vi "PH_Switch.panel.vi"(0 "object ref":refnum<vi>, 5 "error in (no error)":errorcluster) -> (19 "error out":errorcluster)   [LabVIEW 2014, in "PH_Switch.lvlib"]
doc: "By this VI a hardware switch can be monitored and switched. \n\nThe indicators \"FALSE\", \"TRUE\" and \"SWITCH STATE\" show the value of the Beckhoff-Tag: blue indicates bad tag status reference problems, darkgreen false and lightgreen true. If everything is working fine, \"FALSE\" and \"SWITCH STATE\" should show the same value, while \"TRUE\" has the opposite value. The caption of the sensors for \"FALSE\" and \"TRUE\" are taken out of the database. In case of only one or no sensor these GUI elements are not shown at all.\n\nThe oval button switches. It should be in the same state as the \"SWITCH STATE\" indicator. \n\n\"Delete Instance\" disconnects and removes the instance from the PCS.\n\n\nLicense Agreement for this software:\n\nCopyright (C)\nGesellschaft für Schwerionenforschung, GSI\nPlanckstr. 1\n64291 Darmstadt\nGermany\n\nContact: D.Beck@gsi.de \n\nThis program is free software; you can redistribute it and/or modify it under the terms of the GNU General Public License as published by the Free Software Foundation; either version 2 of the license, or (at your option) any later version.\n\nThis program is distributed in the hope that it will be useful, but WITHOUT ANYW ARRANTY; without even the implied warranty of MERCHANTABILITY or FITNESS FOR A PARTICULAR PURPOSE. See the GNU General License for more details (http://www.gnu.org).\n\nGesellschaft für Schwerionenforschung, GSI\nPlanckstr. 1, 64291 Darmstadt, Germany\nFor all questions and ideas contact: M.Richter@gsi.de, H.Brand@gsi.de or D.Beck@gsi.de.\nLast update: 18-DEC-2002"
uses:
  PH_Switch.lvlib
  PH_StatusHandler/PH_StatusHandler.GUI element.ctl
  PH_Switch.GUI Refs.ctl
  CSCore/CSObj/CSObj.lvlib
  CSCore/CSSystem/CSSystemLib/CSSystemLib.lvlib
  PH_Common/PH_Common.lvlib
  PH_PSDBWriter/PH_PSDBWriter.lvlib
  PH_Class/PH_Class.lvlib
  PH_StatusHandler/PH_StatusHandler.lvlib
panel:
  out "Textfield":string="Testtext"
  out "PSDB Status":u32(colorbox)=6618880 caption="PSDB"
  out "Status":T1 caption="Enabling State"
  in  "Exit":bool
  in  "Delete":bool
  in  "Knob":bool
  out "SW STATE":u32(colorbox)
  out "FALSE":u32(colorbox)
  out "TRUE":u32(colorbox)
  # "PCS"
  # "3.40"
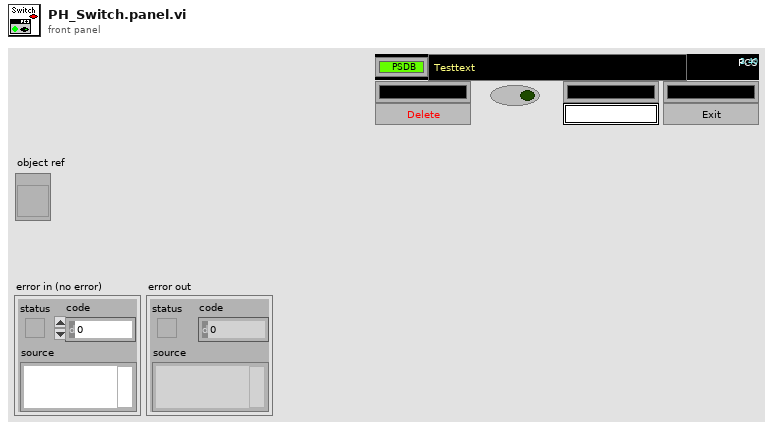
[diagram p1: front panel]
types:
  T1 = typedef "PH_StatusHandler.lvlib/PH_StatusHandler.GUI element.ctl" = u16
  T2 = typedef "PH_Switch.lvlib/PH_Switch.GUI Refs.ctl" = cluster{"true":refnum<vi>, "false":refnum<vi>, "Switch_state":refnum<vi>, "GUI-Knob":refnum<vi>, "Delete":refnum<vi>, "Function Textfield":refnum<vi>}
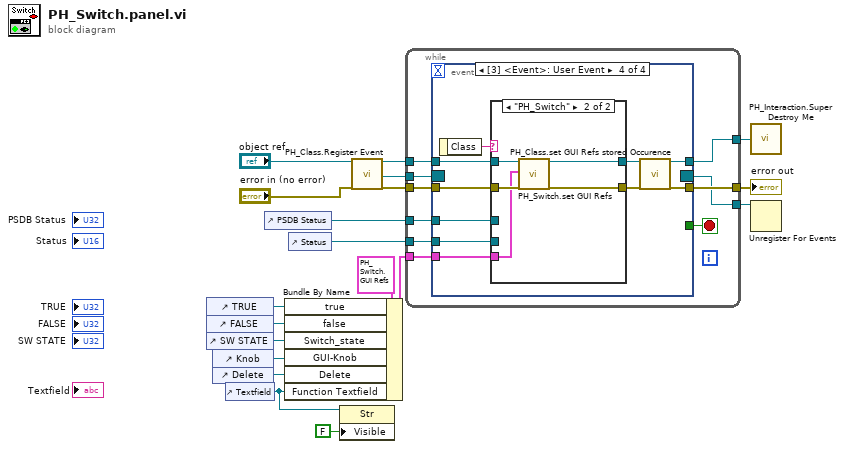
[diagram p0: block diagram]
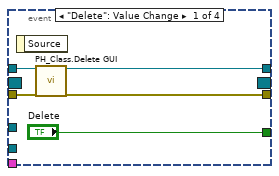
[diagram p2: hidden frame]
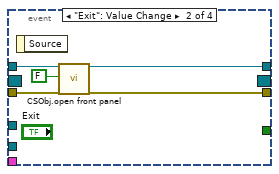
[diagram p3: hidden frame]
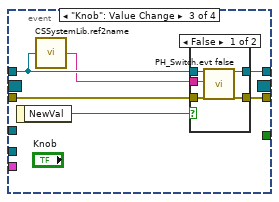
[diagram p4: hidden frame]
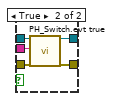
[diagram p5: hidden frame]
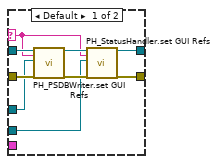
[diagram p6: hidden frame]
diagram:
  n1 = control-ref of="TRUE"() -> (w19:refnum<vi>)
  n2 = control-ref of="FALSE"() -> (w18:refnum<vi>)
  n3 = control-ref of="SW STATE"() -> (w17:refnum<vi>)
  n4 = control-ref of="Knob"() -> (w16:refnum<vi>)
  n5 = control-ref of="Delete"() -> (w15:refnum<vi>)
  n6 = control-ref of="Textfield"() -> (w2:refnum<vi>)
  n7 = control-ref of="PSDB Status"() -> (w9:refnum<vi>)
  n8 = Bundle By Name(cluster=T2 {"true"=refnum, "false"=refnum, "Switch_state"=refnum, "GUI-Knob"=refnum, "Delete"=refnum, "Function Textfield"=refnum} ("GUI Refs"), "true"=w19, "false"=w18, "Switch_state"=w17, "GUI-Knob"=w16, "Delete"=w15, "Function Textfield"=w2) -> (w4:T2)
  n9 = control-ref of="Status"() -> (w1:refnum<vi>)
  n10 = property class="Str"(reference=w2, "Visible"=FALSE) -> ()  [unwired: 1 in, 2 out]
  n11 = call "PH_Class.Register Event.vi"("i ref in"="object ref", "error in (no error)"="error in (no error)") -> ("i ref out"=w12:refnum<vi>, "Event Registration Refnum"=w10:refnum<event-registration>, "error out"=w11:errorcluster)  [unwired: 15 in]
  n12 = while {
    tunnel: w12 -> [w26]
    tunnel: [w25] -> w14
    tunnel: w11 -> [w28]
    tunnel: [w27] -> w13
    tunnel: w10 -> [w23]
    tunnel: w9 -> [w24]
    tunnel: [w21] -> w7
    tunnel: w4 -> [w22]
    tunnel: w1 -> [w20]
    stop <- w29 stop-if-true
    n13 = event shown="[3] <Event>: User Event" {
      selector: w23 -> [_ _ _ _]
      dyn-events: [_ _ _ _] -> w21
      timeout: _ -> [_ _ _ _]
      tunnel: ["Delete" _ _ _] -> w29
      tunnel: w26 -> [w33 w38 w42 w65]
      tunnel: w28 -> [w32 w37 w45 w64]
      tunnel: [w30 w36 w44 w60] -> w27
      tunnel: [w31 w35 w40 w57] -> w25
      tunnel: w24 -> [_ _ _ w63]
      tunnel: w22 -> [_ _ _ w61]
      tunnel: w20 -> [_ _ _ w56]
      event "Delete": Value Change {
        n14 = event-data() -> ()  [unwired: 1 in, 1 out]
        n15 = call "PH_Class.Delete GUI.vi"("VI in"=w33, "error in (no error)"=w32) -> ("VI out"=w31:refnum<vi>, "error out"=w30:errorcluster)  [unwired: 16 in]
      }
      event "Exit": Value Change {
        n16 = event-data() -> ()  [unwired: 1 in, 1 out]
        n17 = call "CSObj.open front panel.vi"("i ref in"=w38, "frontPanelOpen"=FALSE ("front panel open"), "error in (no error)"=w37) -> ("i ref out"=w35:refnum<vi>, "error out"=w36:errorcluster)  [unwired: 15 in]
      }
      event "Knob": Value Change {
        n18 = event-data() -> ("NewVal"=w43:bool)  [unwired: 1 in]
        n19 = call "CSSystemLib.ref2name.vi"("obj refnum"=w42) -> ("name"=w41:string)
        n20 = case shown="False" w43 {
          tunnel: w42 -> [w50 w55]
          tunnel: w45 -> [w49 w54]
          tunnel: [w48 w53] -> w44
          tunnel: w41 -> [w47 w52]
          tunnel: [w46 w51] -> w40
          frame False {
            n21 = call "PH_Switch.evt false.vi"("i ref in"=w50, "Instance"=w47, "error in (no error)"=w49) -> ("i ref out"=w46:refnum<vi>, "error out"=w48:errorcluster)  [unwired: 15 in]
          }
          frame True {
            n22 = call "PH_Switch.evt true.vi"("i ref in"=w55, "Instance"=w52, "error in (no error)"=w54) -> ("i ref out"=w51:refnum<vi>, "error out"=w53:errorcluster)  [unwired: 15 in]
          }
        }
      }
      event User Event {
        n23 = event-data() -> ("Class"=w62:string)  [unwired: 1 in]
        n24 = case shown="\"PH_Switch\"" w62 {
          selector: w62 -> [w67 _]
          tunnel: w65 -> [w74 w79]
          tunnel: [w68 w78] -> w58
          tunnel: w64 -> [w73 w77]
          tunnel: [w70 w76] -> w59
          tunnel: w63 -> [w71 _]
          tunnel: w61 -> [_ w75]
          tunnel: w56 -> [w66 _]
          frame Default {
            n25 = call "PH_PSDBWriter.set GUI Refs.vi"("i ref in"=w74, "Class"=w67, "Ref PSDB Status"=w71, "error in"=w73) -> ("i ref out"=w69:refnum<vi>, "error out"=w72:errorcluster)  [unwired: 14 in]
            n26 = call "PH_StatusHandler.set GUI Refs.vi"("i ref in"=w69, "Class"=w67, "GUI Ref"=w66, "error in (no error)"=w72) -> ("i ref out"=w68:refnum<vi>, "error out"=w70:errorcluster)  [unwired: 14 in]
          }
          frame "PH_Switch" {
            n27 = call "PH_Switch.set GUI Refs.vi"("VI in"=w79, "GUI Refs"=w75, "error in (no error)"=w77) -> ("VI out"=w78:refnum<vi>, "error out"=w76:errorcluster)  [unwired: 15 in]
          }
        }
        n28 = call "PH_Class.set GUI Refs stored Occurence.vi"("i ref in"=w58, "error in (no error)"=w59) -> ("i ref out"=w57:refnum<vi>, "error out"=w60:errorcluster)  [unwired: 16 in]
      }
    }
  }
  "error out" <- w13
  n29 = call "PH_Interaction.Super Destroy Me.vi"("i ref out"=w14) -> ()
  n30 = Unregister For Events(event registration refnum=w7) -> ()  [unwired: 1 in, 1 out]
